vi "Make DLL Param(Read Batch Profile Advance Rsp).vi"(1 "Read Batch Profile Advance Rsp":T2) -> (0 "pRsp":T1)   [LabVIEW 8.6, in "Keyence LJ-V7000.lvlib"]
uses:
  Keyence LJ-V7000.lvlib
  Public/Clusters/Read Batch Profile Advance Rsp.ctl
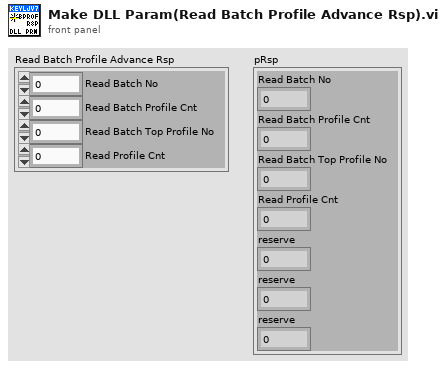
[diagram p1: front panel]
types:
  T1 = cluster{"Read Batch No":u32, "Read Batch Profile Cnt":u32, "Read Batch Top Profile No":u32, "Read Profile Cnt":u8, "reserve":u8, "reserve":u8, "reserve":u8}
  T2 = typedef "Keyence LJ-V7000.lvlib/Read Batch Profile Advance Rsp.ctl" = cluster{"Read Batch No":u32, "Read Batch Profile Cnt":u32, "Read Batch Top Profile No":u32, "Read Profile Cnt":u8}
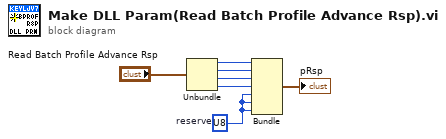
[diagram p0: block diagram]
diagram:
  w2 = u8 ?  # reserve
  n1 = Unbundle("Read Batch Profile Advance Rsp") -> ("Read Batch No"=w6:u32, "Read Batch Profile Cnt"=w5:u32, "Read Batch Top Profile No"=w4:u32, "Read Profile Cnt"=w3:u8)
  n2 = Bundle("Read Batch No"=w6, "Read Batch Profile Cnt"=w5, "Read Batch Top Profile No"=w4, "Read Profile Cnt"=w3, "reserve"=w2, "reserve"=w2, "reserve"=w2) -> (→"pRsp":T1)  [unwired: 1 in]
